vi "AddingChItemsTest.vi"() -> ()   [LabVIEW 2019]
uses:
  SubModules/FPGA Addon Speciality IO/Source/Types/QuadratureEncoder.Measure.Digital.Settings.ctl
  SubModules/FPGA Addon Speciality IO/Source/Types/QuadratureEncoder.Measure.Digital.Measurement.ctl
  SubModules/FPGA Addon Speciality IO/Source/Types/WSS.Generate.Digital.Settings.ctl
  SubModules/FPGA Addon Speciality IO/Source/Types/Static.Measure.Digital.Measurement.ctl
  SubModules/FPGA Addon Speciality IO/Source/Types/Static.Measure.Digital.Settings.ctl
  SubModules/FPGA Addon Speciality IO/Source/Types/Static.Generate.Digital.Settings.ctl
  SubModules/FPGA Addon Speciality IO/Source/Types/PWM.Generate.Digital.Settings.ctl
  SubModules/FPGA Addon Speciality IO/Source/Types/PWM.Measure.Digital.Settings.ctl
  SubModules/FPGA Addon Speciality IO/Source/Types/PWM.Measure.Digital.Measurement.ctl
  SubModules/FPGA Addon Speciality IO/Source/Types/Sine.Generate.Settings.ctl
  SubModules/FPGA Addon Speciality IO/Source/Types/PWM.Measure.Analog.Settings.ctl
  SubModules/FPGA Addon Speciality IO/Source/Types/PWM.Measure.Analog.Measurement.ctl
  <vilib>/Platform/TimedLoop/XDataNode/timing_clust.ctl
  <vilib>/Platform/TimedLoop/XDataNode/nitl_modes.ctl
  <vilib>/Platform/TimedLoop/XDataNode/wakeup.ctl
  <vilib>/rvi/Emulation/niFpgaGetClockAttributes.vi
  <vilib>/rvi/Emulation/niFpgaSctlEmulationGetInTimedLoop.vi
  <vilib>/rvi/Emulation/niFpgaEmulationReportErrorSimple.vi
  <vilib>/rvi/Emulation/niFpgaCriticalErrorInLSC.vi
  <vilib>/rvi/interface/RandomDataEmulation/niFpgaRandomDataHandleErrors.vi
  <vilib>/rvi/DataTransferAndStorage/Container/XNode/niFpgaContainer.xnode
  <vilib>/rvi/interface/RandomDataEmulation/nirviRandomDataFpgaReadWriteTemplate.vi
  <vilib>/Platform/TimedLoop/XDataNode/XDataNode.xnode
  <vilib>/Platform/TimedLoop/XDataNode/XDNodeRunTimeDep.lvlib
  SubModules/FPGA Addon Speciality IO/Source/Speciality FPGA IO.lvlib
panel:
  out "Measure.Analog.Ch6":T1
  in  "Measure.Analog.Ch6.Settings":T2={"ACTIVE EDGE"=TRUE, "TIMEOUT"=40000000, "THRESHOLD"=50.0}
  in  "Generate.Analog.Ch6.Sine.Settings":T3={"AMP"=0.0, "OFFSET"=0.0, "PERIODS/TICKS"=2.4999957531690598e-05}
  out "Measure.Digital.Ch0":T4={"ACTIVE TICKS"=4000, "INACTIVE TICKS"=12000, "ACQ TICKS"=1}
  out "Measure.Digital.Ch1":T4
  in  "Measure.Digital.Ch0.Settings":T5={"ACTIVE EDGE"=TRUE, "TIMEOUT"=40000000}
  in  "Measure.Digital.Ch1.Settings":T5={"ACTIVE EDGE"=FALSE, "TIMEOUT"=40000000}
  in  "Generate.Digital.Ch0.Internal.Settings":T6={"ACTIVE EDGE"=TRUE, "ACTIVE TICKS"=4000, "INACTIVE TICKS"=12000}
  in  "Generate.Digital.Ch1.Internal.Settings":T6={"ACTIVE EDGE"=FALSE, "ACTIVE TICKS"=60000000, "INACTIVE TICKS"=20000000}
  in  "Generate.Digital.Ch2.Internal.Settings":T7={"ACTIVE EDGE"=TRUE, "OUTPUT"=FALSE}
  in  "Measure.Digital.Ch2.Internal.Settings":T8={"ACTIVE EDGE"=TRUE}
  out "Measure.Digital.Ch2":T9
  in  "Generate.Digital.Ch3.Internal.Settings":T7={"ACTIVE EDGE"=TRUE, "OUTPUT"=FALSE}
  in  "Measure.Digital.Ch3.Internal.Settings":T8={"ACTIVE EDGE"=TRUE}
  out "Measure.Digital.Ch3":T9
  in  "Generate.Digital.Ch4.WSS.Settings":T10={"ACTIVE EDGE"=TRUE, "ACTIVE TICKS"=0, "INACTIVE TICKS"=0, "DATA"=0, "SENSOR TYPE"=0}
  out "Generate.Digital.Bit0":bool
  out "Generate.Digital.Bit1":bool
  out "Measurement.Digital.Ch5":T11
  in  "A":bool
  in  "B":bool
  in  "Z":bool
  in  "Measure.Digital.Ch5.QuadEncoder.Settings":T12={"DIRECTION"=0, "RESET VALUE"=0, "A RESET STATE"=TRUE, "B RESET STATE"=TRUE, "Z RESET STATE"=TRUE}
  in  "FXP18.3":fxp<+,18,3>
  out "FXP18.3 out":fxp<+,18,3>
  in  "FXP16.3":fxp<+,16,3>
  out "FXP16.3 out":fxp<+,16,3>
  in  "FXP32.16":fxp<+/-,32,16>
  out "FXP32.16 out":fxp<+/-,32,16>
  in  "FXP27.5":fxp<+/-,27,5>
  out "FXP27.5 out":fxp<+/-,27,5>
  in  "FXP20.5":fxp<+/-,20,5>
  out "FXP20.5 out":fxp<+/-,20,5>
  in  "FXP16.7":fxp<+/-,16,7>
  out "FXP16.7 out":fxp<+/-,16,7>
  out "FXP64.32 out":fxp<+/-,64,32>
  out "FXP32.8 out":fxp<+/-,32,8>
  out "FXP16.5 out":fxp<+/-,16,5>
  out "FXP24.5 out":fxp<+/-,24,5>
  in  "FXP64.32":fxp<+/-,64,32>
  in  "FXP32.8":fxp<+/-,32,8>
  in  "FXP16.5":fxp<+/-,16,5>
  in  "FXP24.5":fxp<+/-,24,5>
  out "Fast timeout":bool
  out "Med timeout":bool
  out "Slow timeout":bool
  in  "I16":i16
  in  "I8":i8
  in  "I64":i64
  in  "I32":i32
  in  "U16":u16
  in  "U8":u8
  in  "U64":u64
  in  "U32":u32
  in  "SGL":sgl
  in  "Boolean":bool
  out "I16 out":i16
  out "I8 out":i8
  out "I64 out":i64
  out "I32 out":i32
  out "U16 out":u16
  out "U8 out":u8
  out "U64 out":u64
  out "U32 out":u32
  out "SGL out":sgl
  out "Boolean out":bool
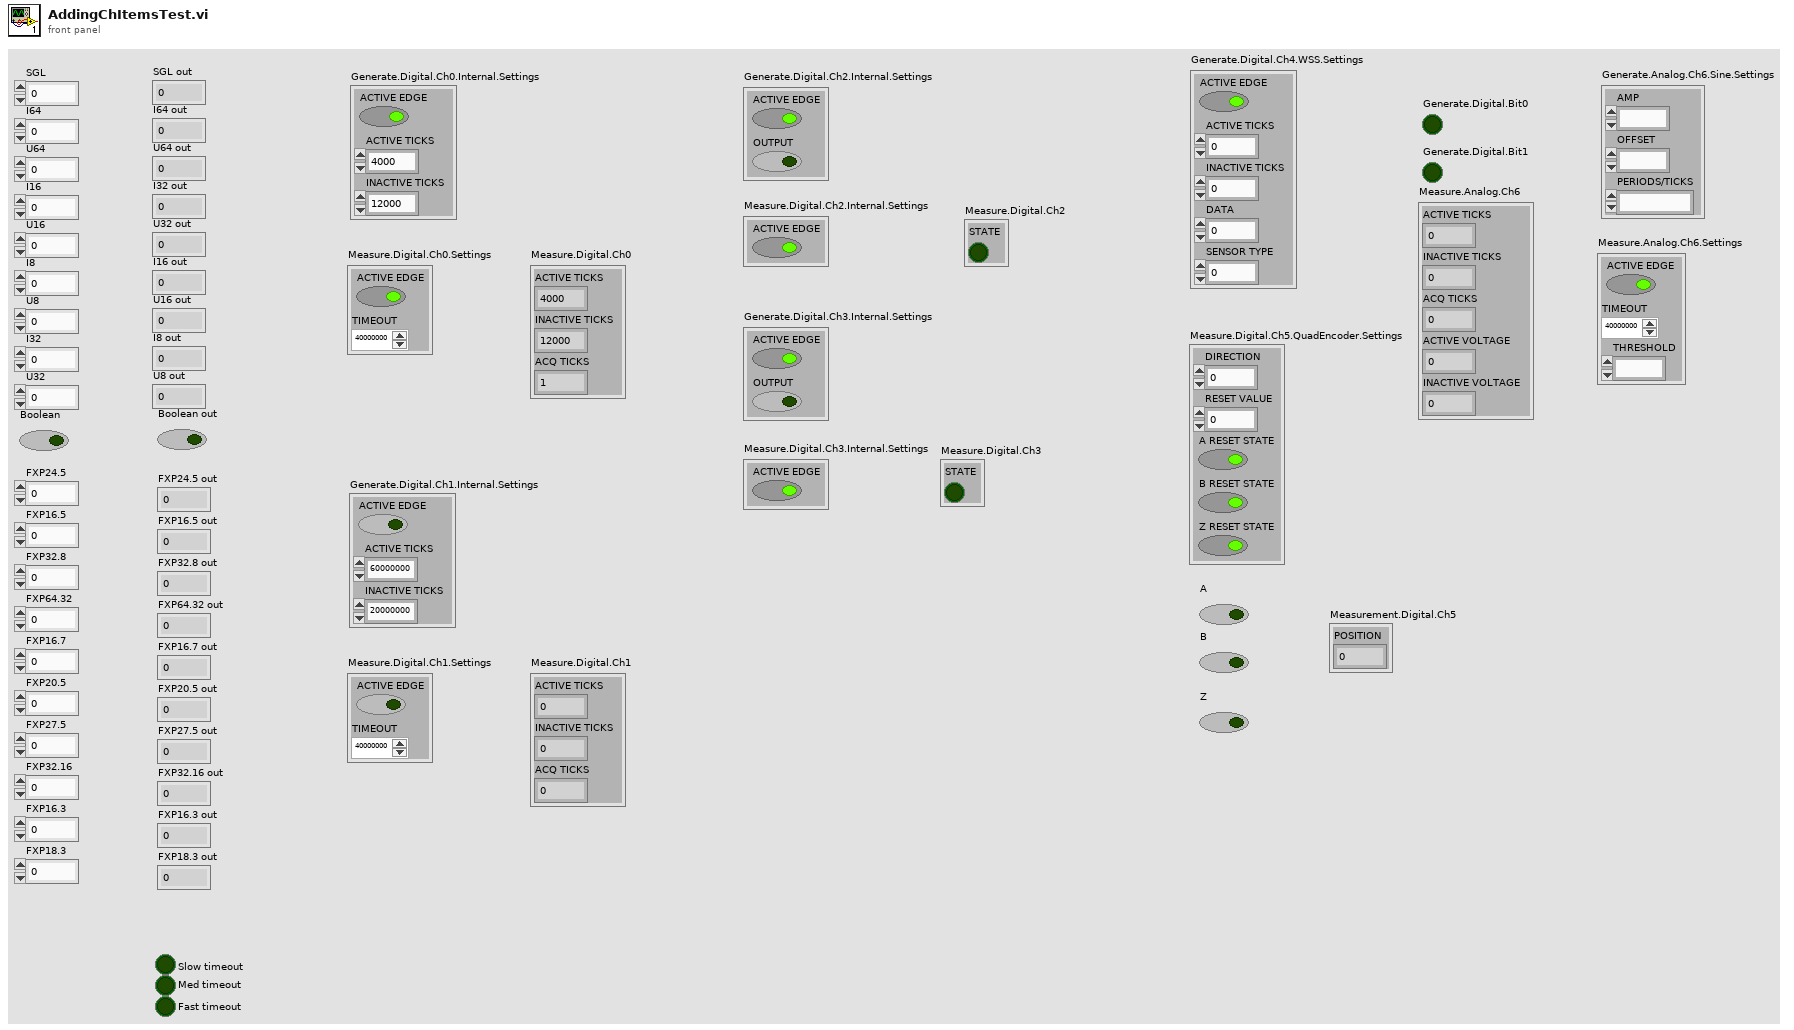
[diagram p1: front panel]
types:
  T1 = typedef "Speciality FPGA IO.lvlib/PWM.Measure.Analog.Measurement.ctl" = cluster{"ACTIVE TICKS":u32, "INACTIVE TICKS":u32, "ACQ TICKS":u32, "ACTIVE VOLTAGE":fxp<+/-,32,8>, "INACTIVE VOLTAGE":fxp<+/-,32,8>}
  T2 = typedef "Speciality FPGA IO.lvlib/PWM.Measure.Analog.Settings.ctl" = cluster{"ACTIVE EDGE":bool, "TIMEOUT":u32, "THRESHOLD":fxp<+/-,32,8>}
  T3 = typedef "Speciality FPGA IO.lvlib/Sine.Generate.Settings.ctl" = cluster{"AMP":fxp<+/-,32,8>, "OFFSET":fxp<+/-,32,8>, "PERIODS/TICKS":fxp<+,32,0>}
  T4 = typedef "Speciality FPGA IO.lvlib/PWM.Measure.Digital.Measurement.ctl" = cluster{"ACTIVE TICKS":u32, "INACTIVE TICKS":u32, "ACQ TICKS":u32}
  T5 = typedef "Speciality FPGA IO.lvlib/PWM.Measure.Digital.Settings.ctl" = cluster{"ACTIVE EDGE":bool, "TIMEOUT":u32}
  T6 = typedef "Speciality FPGA IO.lvlib/PWM.Generate.Digital.Settings.ctl" = cluster{"ACTIVE EDGE":bool, "ACTIVE TICKS":u32, "INACTIVE TICKS":u32}
  T7 = typedef "Speciality FPGA IO.lvlib/Static.Generate.Digital.Settings.ctl" = cluster{"ACTIVE EDGE":bool, "OUTPUT":bool}
  T8 = typedef "Speciality FPGA IO.lvlib/Static.Measure.Digital.Settings.ctl" = cluster{"ACTIVE EDGE":bool}
  T9 = typedef "Speciality FPGA IO.lvlib/Static.Measure.Digital.Measurement.ctl" = cluster{"STATE":bool}
  T10 = typedef "Speciality FPGA IO.lvlib/WSS.Generate.Digital.Settings.ctl" = cluster{"ACTIVE EDGE":bool, "ACTIVE TICKS":u32, "INACTIVE TICKS":u32, "DATA":u8, "SENSOR TYPE":u8}
  T11 = typedef "Speciality FPGA IO.lvlib/QuadratureEncoder.Measure.Digital.Measurement.ctl" = cluster{"POSITION":i32}
  T12 = typedef "Speciality FPGA IO.lvlib/QuadratureEncoder.Measure.Digital.Settings.ctl" = cluster{"DIRECTION":u8, "RESET VALUE":i32, "A RESET STATE":bool, "B RESET STATE":bool, "Z RESET STATE":bool}
  T13 = typedef "XDNodeRunTimeDep.lvlib/timing_clust.ctl" = cluster{"Expected End [f-1]":u64, "Actual End [f-1]":u64, "Finished Late? [f-1]":bool, "Expected End [i-1]":u64, "Actual End [i-1]":u64, "Finished Late? [i-1]":bool, "Expected Start [i]":u64, "Actual Start [i]":u64, "Expected Start [f]":u64, "Actual Start [f]":u64, "Source Name":string, "Structure Name":string, "Period":i64, "Deadline":i64, "Offset":i64, "Start":i64, "Priority":i32, "Timeout":i32, "Mode":T14, "Wakeup Reason":T15, "Error":errorcluster, "Source Type":string, "Secondary Source Type":string, "Global End Time":u64, "Global Start Time":u64, "Frame Duration":u64, "Iteration Duration":u64, "Assigned CPU":i32, "I/O Scan Engine Mode":u32}
  T14 = typedef "XDNodeRunTimeDep.lvlib/nitl_modes.ctl" = enum32{"No Change", "Process missed periods, maintain original phase", "Discard missed periods, maintain original phase", "Process missed periods, ignore original phase", "Discard missed periods, ignore original phase"}
  T15 = typedef "XDNodeRunTimeDep.lvlib/wakeup.ctl" = enum32{"Normal", "Aborted", "Asynchronous wakeup", "Timing source error", "Timed loop error", "Timeout"}
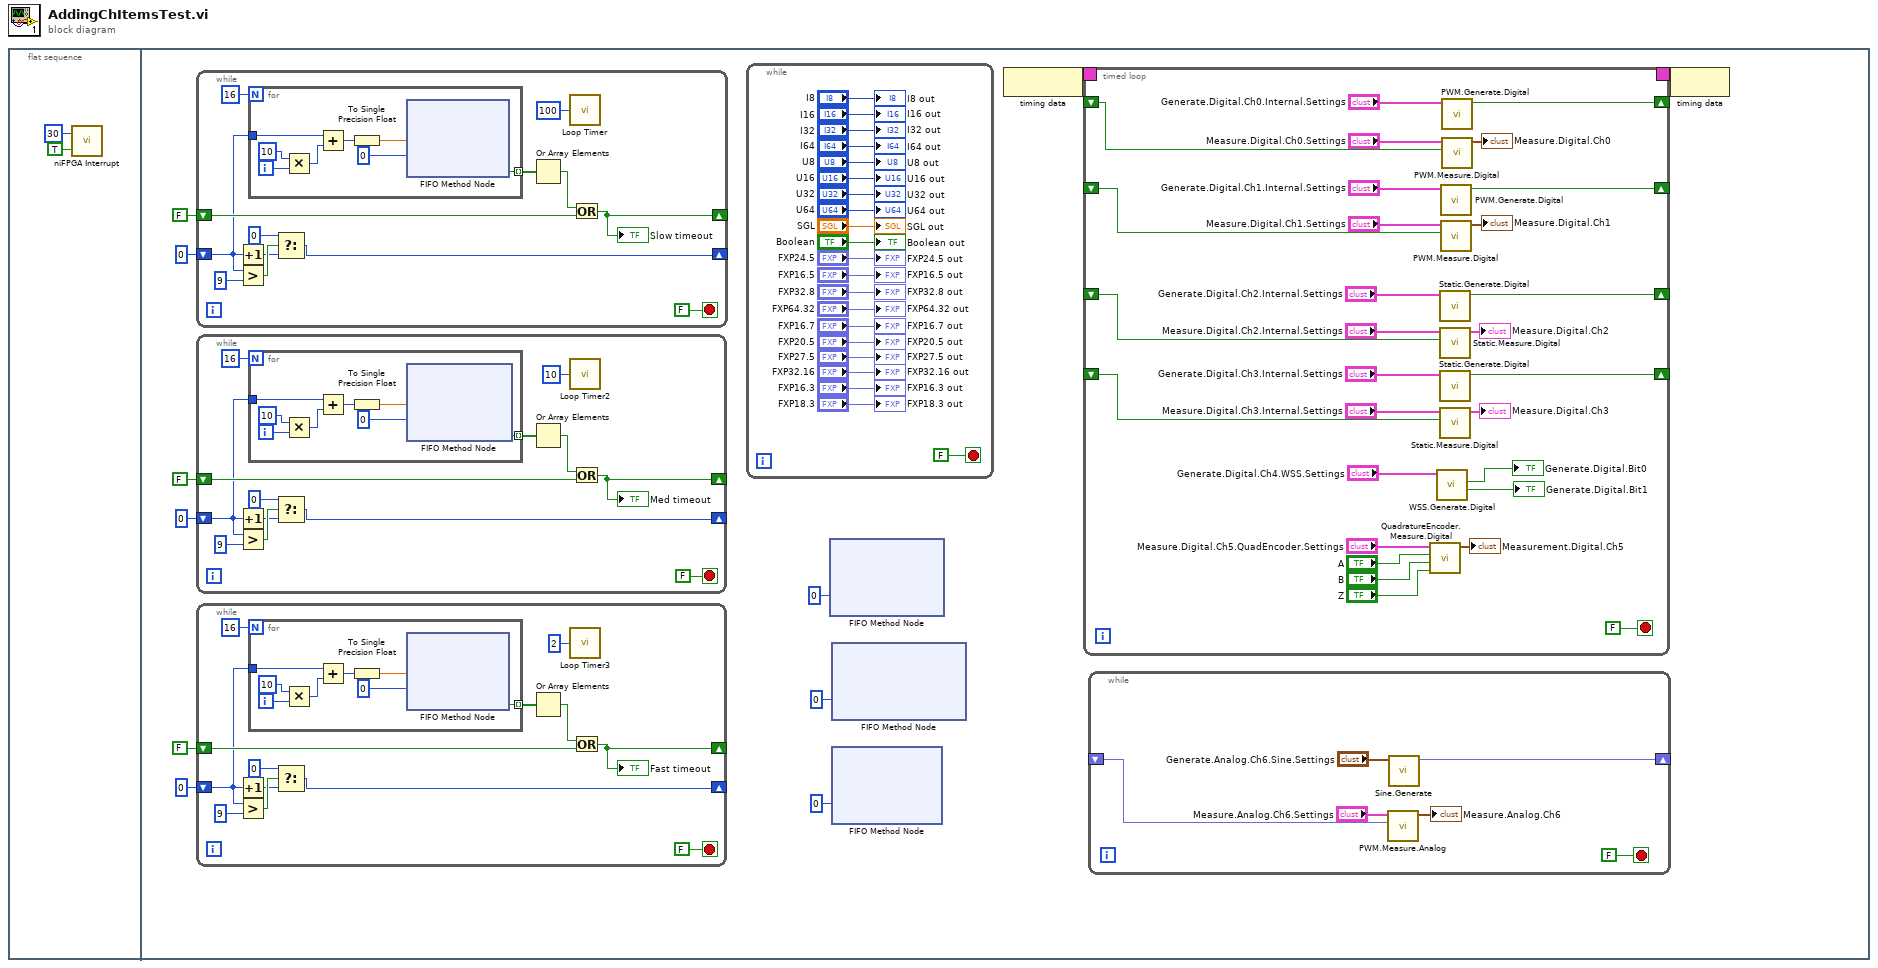
[diagram p0: block diagram]
diagram:
  n1 = flat-sequence {
    frame #0 {
      n2 = call <vilib>:"niFPGA Interrupt.vi"("Wait Until Cleared (F)"=TRUE, "IRQ Number (0)"=u8 30) -> ()  [unwired: 1 in]
    }
    frame #1 {
      n3 = while {
        shift-right: [w102] -> _
        shift-left: 0 ("t") -> [w95]
        shift-right: [w96] -> _
        shift-left: FALSE -> [w97]
        stop <- FALSE stop-if-true
        n4 = Increment(x=w95) -> (x+1=w100:i32)
        n5 = Greater?(x=w95, y=9) -> (0:w106:bool)
        n6 = for {
          N: 16 -> [_]
          tunnel: w95 -> [w115]
          tunnel: [w108] -> w99 mode=indexing
          i -> [w114]
          n7 = Multiply(x=10, y=w114) -> (x*y=w112:i32)
          n8 = Add(x=w115, y=w112) -> (x+y=w111:i32)
          n9 = To Single Precision Float(number=w111) -> (single precision float=w110:sgl)
          n10 = xnode ("FIFO Method Node")("Element"=w110, "Timeout"=0) -> ("Timed Out?"=w108:bool)  [unwired: 1 in, 1 out]
        }
        n11 = Select(t=0, s=w106, f=w100) -> (s? t:f=w102:i32)
        n12 = Or Array Elements(Boolean array=w99) -> (logical OR=w98:bool)
        n13 = call "Loop Timer"("Count(uSec)"=u32 100) -> ()  [unwired: 1 out]
        n14 = Or(x=w98, y=w97) -> (x .or. y?=w96:bool)
        "Slow timeout" <- w96
      }
      n15 = while {
        shift-right: [w81] -> _
        shift-left: 0 ("t") -> [w74]
        shift-right: [w75] -> _
        shift-left: FALSE -> [w76]
        stop <- FALSE stop-if-true
        n16 = Increment(x=w74) -> (x+1=w79:i32)
        n17 = Greater?(x=w74, y=9) -> (0:w85:bool)
        n18 = for {
          N: 16 -> [_]
          tunnel: w74 -> [w94]
          tunnel: [w87] -> w78 mode=indexing
          i -> [w93]
          n19 = Multiply(x=10, y=w93) -> (x*y=w91:i32)
          n20 = Add(x=w94, y=w91) -> (x+y=w90:i32)
          n21 = To Single Precision Float(number=w90) -> (single precision float=w89:sgl)
          n22 = xnode ("FIFO Method Node")("Element"=w89, "Timeout"=0) -> ("Timed Out?"=w87:bool)  [unwired: 1 in, 1 out]
        }
        n23 = Select(t=0, s=w85, f=w79) -> (s? t:f=w81:i32)
        n24 = Or Array Elements(Boolean array=w78) -> (logical OR=w77:bool)
        n25 = call "Loop Timer2"("Count(uSec)"=u32 10) -> ()  [unwired: 1 out]
        n26 = Or(x=w77, y=w76) -> (x .or. y?=w75:bool)
        "Med timeout" <- w75
      }
      n27 = while {
        shift-right: [w60] -> _
        shift-left: 0 ("t") -> [w53]
        shift-right: [w54] -> _
        shift-left: FALSE -> [w55]
        stop <- FALSE stop-if-true
        n28 = Increment(x=w53) -> (x+1=w58:i32)
        n29 = Greater?(x=w53, y=9) -> (0:w64:bool)
        n30 = for {
          N: 16 -> [_]
          tunnel: w53 -> [w73]
          tunnel: [w66] -> w57 mode=indexing
          i -> [w72]
          n31 = Multiply(x=10, y=w72) -> (x*y=w70:i32)
          n32 = Add(x=w73, y=w70) -> (x+y=w69:i32)
          n33 = To Single Precision Float(number=w69) -> (single precision float=w68:sgl)
          n34 = xnode ("FIFO Method Node")("Element"=w68, "Timeout"=0) -> ("Timed Out?"=w66:bool)  [unwired: 1 in, 1 out]
        }
        n35 = Select(t=0, s=w64, f=w58) -> (s? t:f=w60:i32)
        n36 = Or Array Elements(Boolean array=w57) -> (logical OR=w56:bool)
        n37 = call "Loop Timer3"("Count(uSec)"=u32 2) -> ()  [unwired: 1 out]
        n38 = Or(x=w56, y=w55) -> (x .or. y?=w54:bool)
        "Fast timeout" <- w54
      }
      n39 = while {
        stop <- FALSE stop-if-true
        "I16 out" <- "I16"
        "I8 out" <- "I8"
        "I64 out" <- "I64"
        "I32 out" <- "I32"
        "U16 out" <- "U16"
        "U8 out" <- "U8"
        "U64 out" <- "U64"
        "U32 out" <- "U32"
        "SGL out" <- "SGL"
        "Boolean out" <- "Boolean"
        "FXP24.5 out" <- "FXP24.5"
        "FXP16.5 out" <- "FXP16.5"
        "FXP32.8 out" <- "FXP32.8"
        "FXP64.32 out" <- "FXP64.32"
        "FXP16.7 out" <- "FXP16.7"
        "FXP20.5 out" <- "FXP20.5"
        "FXP27.5 out" <- "FXP27.5"
        "FXP32.16 out" <- "FXP32.16"
        "FXP16.3 out" <- "FXP16.3"
        "FXP18.3 out" <- "FXP18.3"
      }
      n40 = xnode ("FIFO Method Node")("Timeout"=0) -> ()  [unwired: 1 in, 3 out]
      n41 = xnode ("FIFO Method Node")("Timeout"=0) -> ()  [unwired: 1 in, 3 out]
      n42 = xnode ("FIFO Method Node")("Timeout"=0) -> ()  [unwired: 1 in, 3 out]
      n43 = node-c288() -> (w7:T13)
      n44 = timed-loop {
        timing: w7 -> [_]
        timing-out: [_] -> w6
        shift-right: [w47] -> _
        shift-left: _ -> [w46]
        shift-right: [w45] -> _
        shift-left: _ -> [w44]
        shift-right: [w37] -> _
        shift-left: _ -> [w35]
        shift-right: [w28] -> _
        shift-left: _ -> [w30]
        stop <- FALSE stop-if-true
        n45 = call "QuadratureEncoder.Measure.Digital.vi"("Z"="Z", "B"="B", "A"="A", "Settings"="Measure.Digital.Ch5.QuadEncoder.Settings") -> ("Measurement"=→"Measurement.Digital.Ch5":T11)  [unwired: 7 in]
        n46 = call "WSS.Generate.Digital.vi"("Settings"="Generate.Digital.Ch4.WSS.Settings") -> ("Bit1"=→"Generate.Digital.Bit1":bool, "Bit0"=→"Generate.Digital.Bit0":bool)  [unwired: 8 in, 1 out]
        n47 = call "Static.Generate.Digital.vi"("Settings"="Generate.Digital.Ch2.Internal.Settings") -> ("Output"=w37:bool)  [unwired: 10 in]
        n48 = call "Static.Measure.Digital.vi"("State"=w35, "Settings"="Measure.Digital.Ch2.Internal.Settings") -> ("Measurement"=→"Measure.Digital.Ch2":T9)  [unwired: 9 in]
        n49 = call "Static.Generate.Digital.vi"("Settings"="Generate.Digital.Ch3.Internal.Settings") -> ("Output"=w28:bool)  [unwired: 10 in]
        n50 = call "Static.Measure.Digital.vi"("State"=w30, "Settings"="Measure.Digital.Ch3.Internal.Settings") -> ("Measurement"=→"Measure.Digital.Ch3":T9)  [unwired: 9 in]
        n51 = call "PWM.Generate.Digital.vi"("Settings"="Generate.Digital.Ch1.Internal.Settings") -> ("Output"=w47:bool)  [unwired: 10 in]
        n52 = call "PWM.Measure.Digital.vi"("State"=w46, "Settings"="Measure.Digital.Ch1.Settings") -> ("Measurement"=→"Measure.Digital.Ch1":T4)  [unwired: 8 in, 1 out]
        n53 = call "PWM.Generate.Digital.vi"("Settings"="Generate.Digital.Ch0.Internal.Settings") -> ("Output"=w45:bool)  [unwired: 10 in]
        n54 = call "PWM.Measure.Digital.vi"("State"=w44, "Settings"="Measure.Digital.Ch0.Settings") -> ("Measurement"=→"Measure.Digital.Ch0":T4)  [unwired: 8 in, 1 out]
      }
      n55 = while {
        shift-right: [w15] -> _
        shift-left: _ -> [w14]
        stop <- FALSE stop-if-true
        n56 = call "PWM.Measure.Analog.vi"("PWM"=w14, "Settings"="Measure.Analog.Ch6.Settings") -> ("Measurement"=→"Measure.Analog.Ch6":T1)  [unwired: 8 in, 1 out]
        n57 = call "Sine.Generate.vi"("Settings"="Generate.Analog.Ch6.Sine.Settings") -> ("Output"=w15:fxp<+/-,32,8>)  [unwired: 10 in]
      }
      n58 = node-c288(w6) -> ()
    }
  }
